vi "Voltage_Current_Sweep.vi"() -> ()   [LabVIEW 2016]
uses:
  <instrlib>/Keithley 24XX/Public/Data/Read (Single Point).vi
  <instrlib>/Keithley 24XX/Keithley 24XX.lvlib
panel:
  in  "Tab Control":enum32{"Voltage", "Current"}(tab)
  in  "Start (V)":dbl
  in  "End (V)":dbl=100.0
  in  "Compliance (V)":dbl=0.1
  in  "Interval (V)":dbl=100.0
  in  "Start (mA)":dbl
  in  "End (mA)":dbl=100.0
  in  "Compliance (A)":dbl=0.1
  in  "Interval (mA)":dbl=100.0
  in  "file (use dialog)":path
  in  "2wire(F)/4wire(T)":bool=TRUE
  out "IV":cluster{dbl[], dbl[]}(graph)
  out "Voltage":sgl=100.0186
  out "Current":sgl=-1.469503e-10
  out "Resistance":sgl=-680628800000.0
  in  "Delay Time (s)":dbl=1.0
  out "VR":cluster{dbl[], dbl[]}(graph)
  out "IR":cluster{dbl[], dbl[]}(graph)
  in  "Enable Resistance Auto Range (T:Enable)":bool=TRUE
  in  "Enable Current Auto Range (T:Enable)":bool=TRUE
  in  "Enable Voltage Auto Range (T:Enable)":bool=TRUE
  in  "Resistance Manual Range (1.0)":dbl=1.0
  in  "Current Manual Range (1.0)":dbl=1.0
  in  "Voltage Manual Range (1.0)":dbl=1.0
  in  "Serial Configuration":T1={"Baud Rate"=9600, "Parity"=0, "Data Bits"=8, "Stop Bits"=10, "Flow Control"=0} {"Flow Control" items=["None", "XON/XOFF", "RTS/CTS", "XON/XOFF & RTS/CTS", "DTR/DSR", "XON/XOFF & DTR/DSR"]; "Stop Bits" items=["1.0"=10, "1.5"=15, "2.0"=20]; "Data Bits" items=["7"=7, "8"=8]; "Parity" items=["None", "Odd", "Even", "Mark", "Space"]; "Baud Rate" items=["300"=300, "600"=600, "1200"=1200, "2400"=2400, "4800"=4800, "9600"=9600, "19200"=19200]}
  in  "VISA resource name":refnum<visa-resource-name>="COM5"
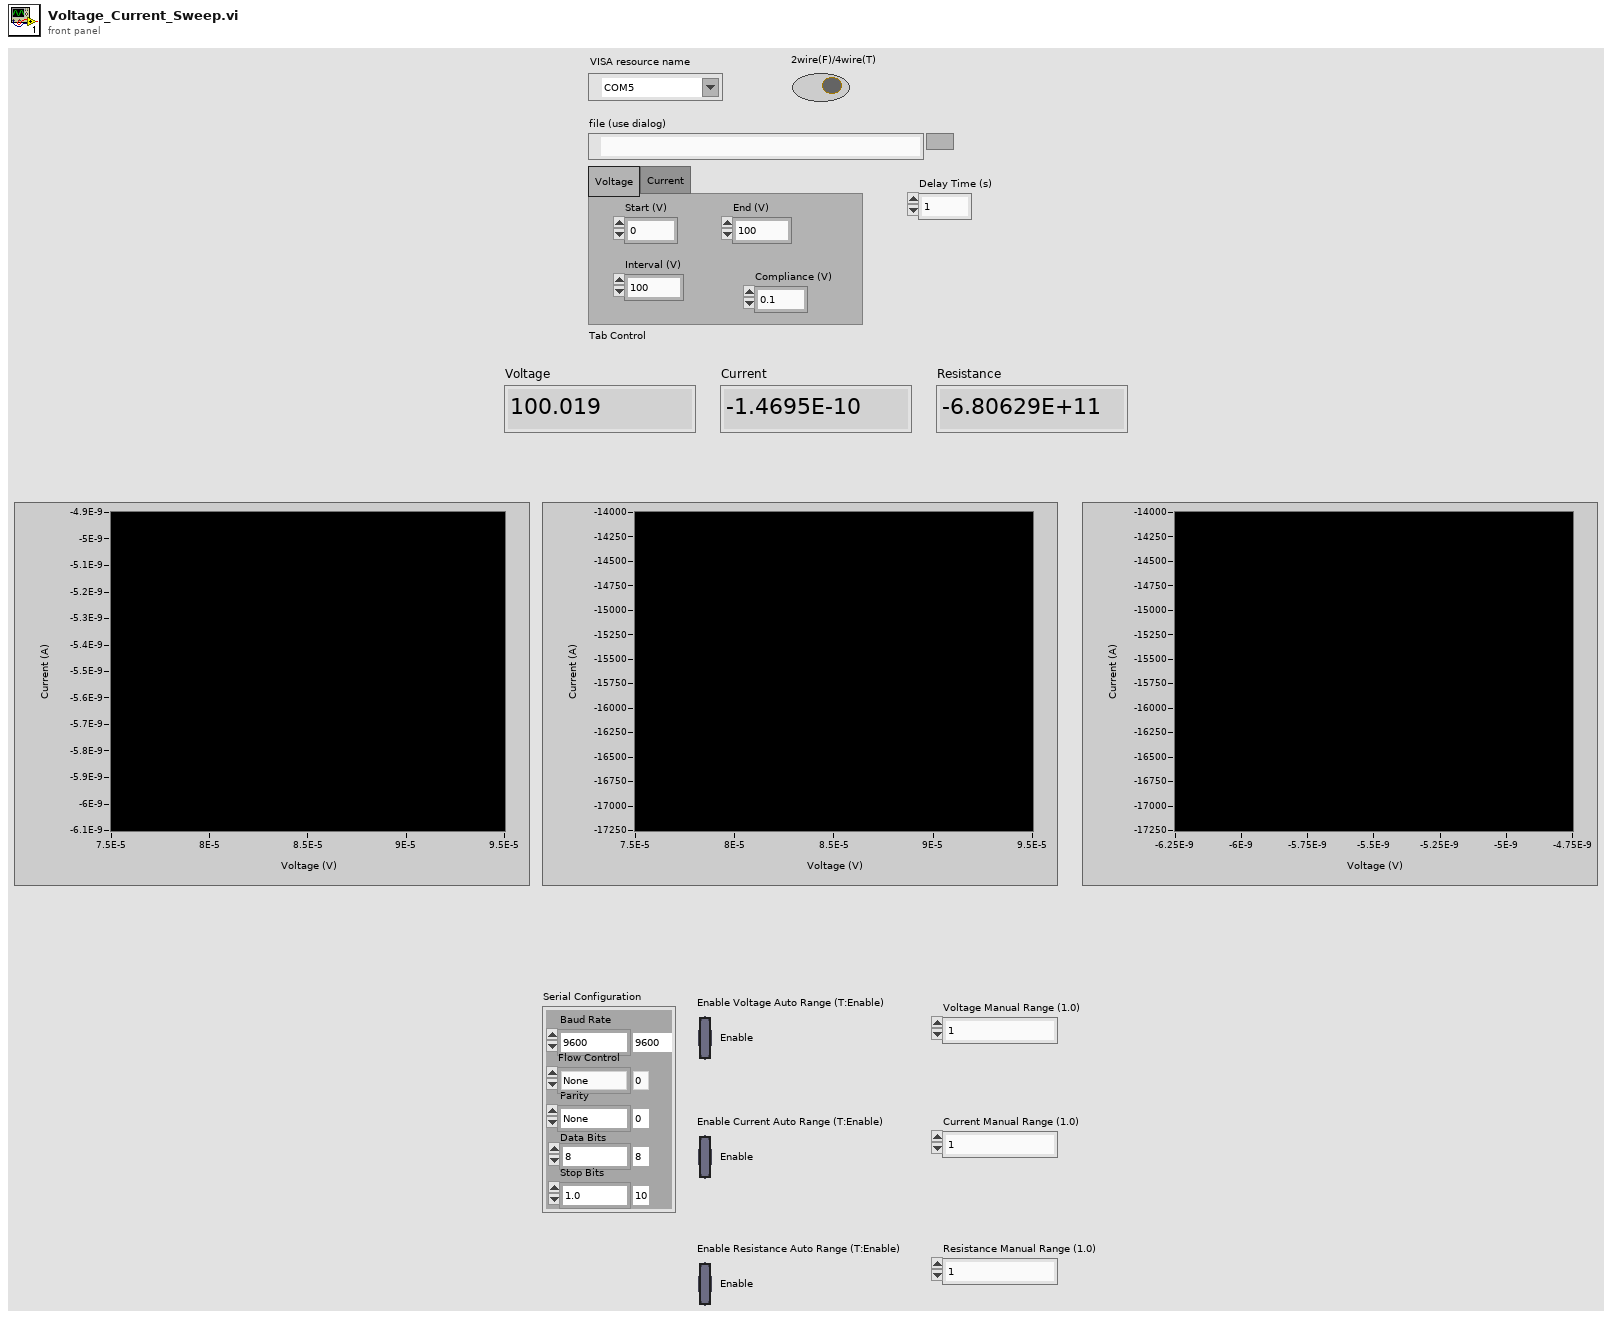
[diagram p1: front panel]
types:
  T1 = cluster{"Baud Rate":u32, "Parity":u16, "Data Bits":u16, "Stop Bits":u16, "Flow Control":u16}
  T2 = enum16{"open", "replace", "create", "open or create", "replace or create", "replace or create with confirmation"}
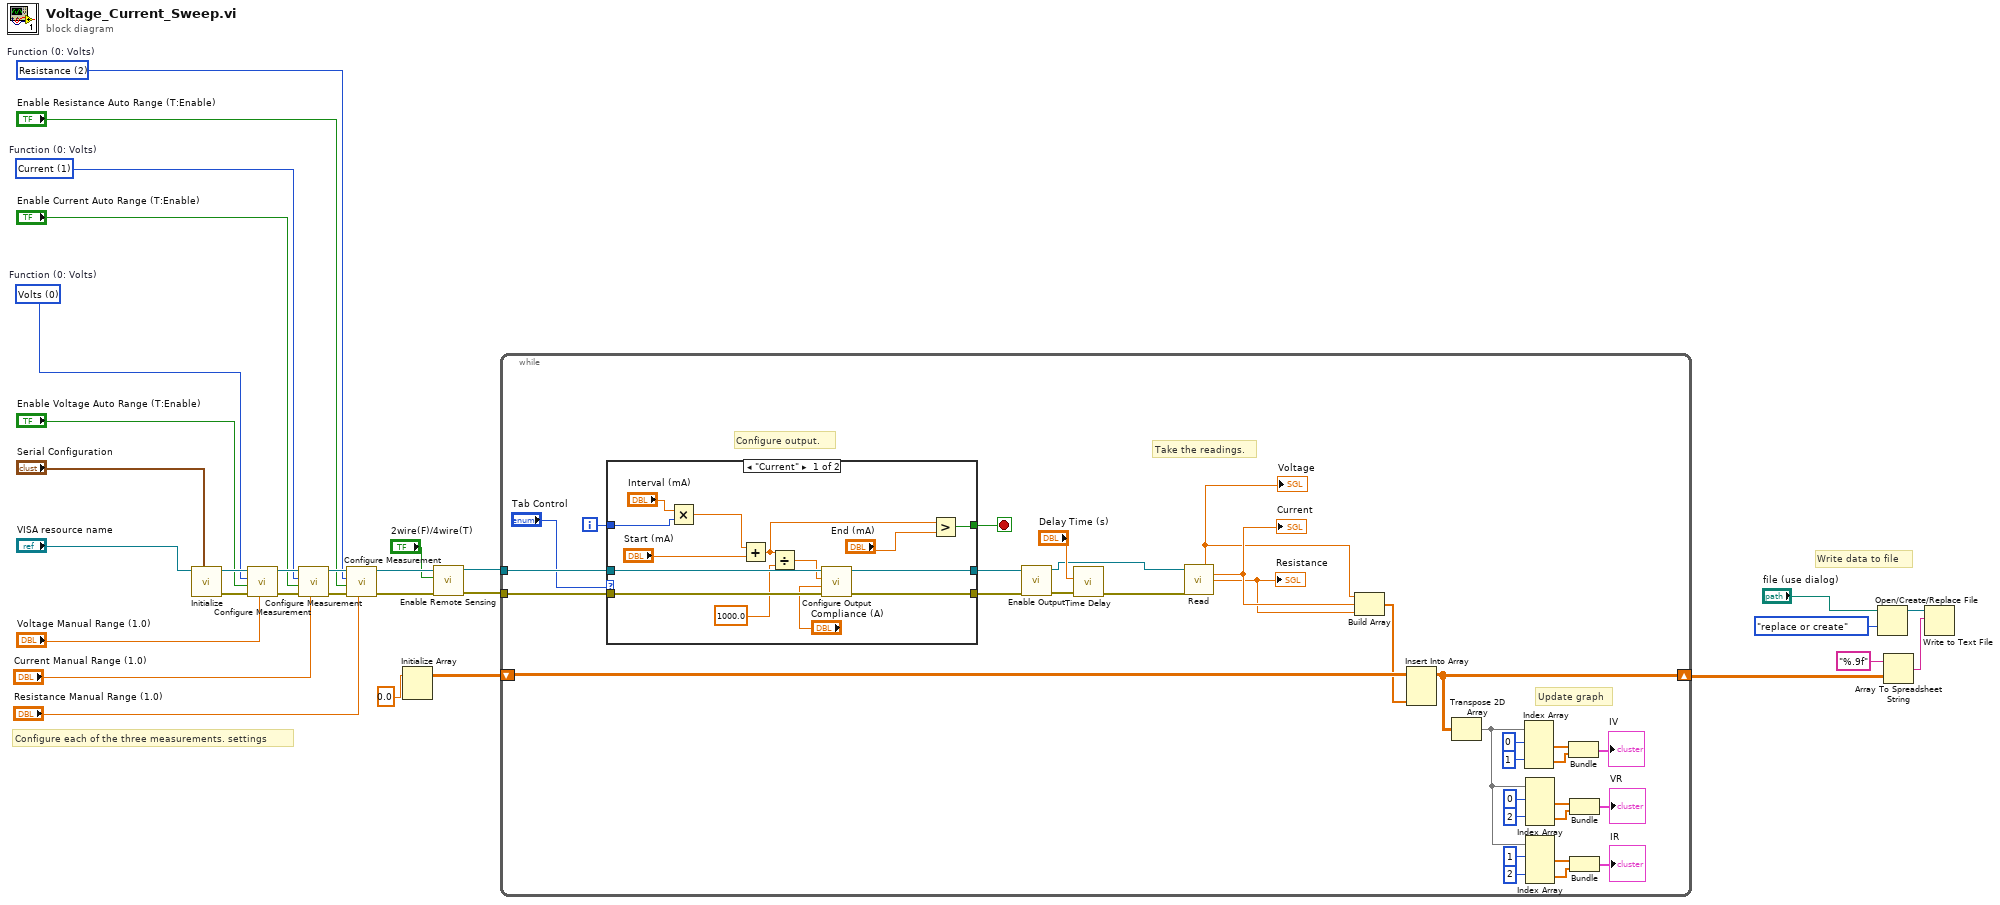
[diagram p0: block diagram]
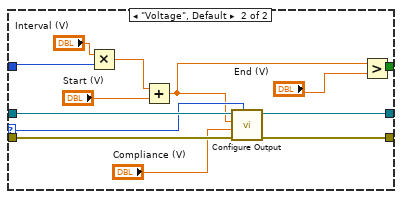
[diagram p2: hidden frame]
diagram:
  w20 = u16 2 items=["Volts", "Current", "Resistance"]  # Function (0: Volts)
  w21 = u16 1 items=["Volts", "Current", "Resistance"]  # Function (0: Volts)
  w22 = u16 0 items=["Volts", "Current", "Resistance"]  # Function (0: Volts)
  # "Write data to file"
  # "Configure each of the three measurements. settings"
  n1 = call <instrlib>:"Initialize.vi"("Serial Configuration"="Serial Configuration", "VISA resource name"="VISA resource name") -> ("error out"=w27:errorcluster, "VISA resource name out"=w28:refnum<visa-resource-name>)  [unwired: 8 in]
  n2 = call <instrlib>:"Configure Measurement.vi"("Manual Range (1.0)"="Voltage Manual Range (1.0)", "error in (no error)"=w27, "Enable Auto Range (T:Enable)"="Enable Voltage Auto Range (T:Enable)", "Function (0: Volts)"=w22, "VISA resource name"=w28) -> ("error out"=w25:errorcluster, "VISA resource name out"=w26:refnum<visa-resource-name>)  [unwired: 5 in]
  n3 = call <instrlib>:"Configure Measurement.vi"("Manual Range (1.0)"="Current Manual Range (1.0)", "error in (no error)"=w25, "Enable Auto Range (T:Enable)"="Enable Current Auto Range (T:Enable)", "Function (0: Volts)"=w21, "VISA resource name"=w26) -> ("error out"=w24:errorcluster, "VISA resource name out"=w23:refnum<visa-resource-name>)  [unwired: 5 in]
  n4 = call <instrlib>:"Configure Measurement.vi"("Manual Range (1.0)"="Resistance Manual Range (1.0)", "error in (no error)"=w24, "Enable Auto Range (T:Enable)"="Enable Resistance Auto Range (T:Enable)", "Function (0: Volts)"=w20, "VISA resource name"=w23) -> ("error out"=w9:errorcluster, "VISA resource name out"=w10:refnum<visa-resource-name>)  [unwired: 5 in]
  n5 = Initialize Array(0.0 ("element")) -> (w11:dbl[][])  [unwired: 2 in]
  n6 = call <instrlib>:"Enable Remote Sensing.vi"("error in (no error)"=w9, "Enable Remote Sensing (T: Enable)"="2wire(F)/4wire(T)", "VISA resource name"=w10) -> ("error out"=w7:errorcluster, "VISA resource name out"=w8:refnum<visa-resource-name>)  [unwired: 7 in]
  n7 = while {
    tunnel: w7 -> [w62]
    tunnel: w8 -> [w63]
    shift-right: [w57] -> w13
    shift-left: w11 -> [w61]
    i -> [w31]
    stop <- w33 stop-if-true
    # "Configure output."
    # "Update graph"
    # "Take the readings."
    n8 = case shown="\"Current\"" "Tab Control" {
      selector: "Tab Control" -> [_ w83]
      tunnel: w63 -> [w77 w90]
      tunnel: w62 -> [w76 w89]
      tunnel: [w74 w87] -> w50
      tunnel: [w73 w86] -> w48
      tunnel: [w69 w84] -> w33
      tunnel: w31 -> [w66 w80]
      frame "Current" {
        n9 = Multiply(x="Interval (mA)", y=w66) -> (x*y=w65:dbl)
        n10 = Add(x=w65, y="Start (mA)") -> (x+y=w68:dbl)
        n11 = Divide(x=w68, y=1000.0) -> (x/y=w70:dbl)
        n12 = call <instrlib>:"Configure Output.vi"("error in (no error)"=w76, "Compliance  Level (0.1)"="Compliance (A)", "Output Level (0)"=w70, "VISA resource name"=w77) -> ("error out"=w73:errorcluster, "VISA resource name out"=w74:refnum<visa-resource-name>)  [unwired: 6 in]
        n13 = Greater?(x=w68, y="End (mA)") -> (0:w69:bool)
      }
      frame "Voltage", Default {
        n14 = Multiply(x="Interval (V)", y=w80) -> (x*y=w79:dbl)
        n15 = Add(x=w79, y="Start (V)") -> (x+y=w78:dbl)
        n16 = call <instrlib>:"Configure Output.vi"("Source Mode  (0: Voltage)"=w83, "error in (no error)"=w89, "Compliance  Level (0.1)"="Compliance (V)", "Output Level (0)"=w78, "VISA resource name"=w90) -> ("error out"=w86:errorcluster, "VISA resource name out"=w87:refnum<visa-resource-name>)  [unwired: 5 in]
        n17 = Greater?(x=w78, y="End (V)") -> (0:w84:bool)
      }
    }
    n18 = call <instrlib>:"Enable Output.vi"("error in (no error)"=w48, "VISA resource name"=w50) -> ("error out"=w47:errorcluster, "VISA resource name out"=w49:refnum<visa-resource-name>)  [unwired: 8 in]
    n19 = call "Time Delay"("error in (no error)"=w47, "Delay Time (s)"="Delay Time (s)") -> ("error out"=w53:errorcluster)  [unwired: 9 in]
    n20 = call-poly <instrlib>:"Read.vi"("VISA resource name"=w49, "error in (no error)"=w53) -> ("Voltage"=w54:sgl, "Current"=w55:sgl, "Resistance"=w51:sgl)  [unwired: 7 in, 4 out]
    "Voltage" <- w54
    "Current" <- w55
    "Resistance" <- w51
    n21 = Build Array(w54, w55, w51) -> (w56:sgl[])
    n22 = Insert Into Array(array=w61, new element=w56) -> (w57:dbl[][])  [unwired: 2 in]
    n23 = Transpose 2D Array(2D array=w57) -> (transposed array=w34:dbl[][])
    n24 = Index Array(array=w34, index (row) #1=0 ("index (row)"), index (row) #2=1 ("index (row)")) -> (element #1=w59:dbl[], element #2=w60:dbl[])  [unwired: 2 in]
    n25 = Index Array(array=w34, index (row) #1=0 ("index (row)"), index (row) #2=2 ("index (row)")) -> (element #1=w43:dbl[], element #2=w44:dbl[])  [unwired: 2 in]
    n26 = Index Array(array=w34, index (row) #1=1 ("index (row)"), index (row) #2=2 ("index (row)")) -> (element #1=w38:dbl[], element #2=w39:dbl[])  [unwired: 2 in]
    n27 = Bundle(w59, w60) -> (→"IV":cluster{dbl[], dbl[]})  [unwired: 1 in]
    n28 = Bundle(w43, w44) -> (→"VR":cluster{dbl[], dbl[]})  [unwired: 1 in]
    n29 = Bundle(w38, w39) -> (→"IR":cluster{dbl[], dbl[]})  [unwired: 1 in]
  }
  n30 = Open/Create/Replace File(file path (use dialog)="file (use dialog)", operation (0:open)=T2."replace or create") -> (refnum out=w2:refnum<file>)  [unwired: 4 in, 2 out]
  n31 = Array To Spreadsheet String(array=w13, 3:"%.9f" ("format string")) -> (spreadsheet string=w5:string)  [unwired: 1 in]
  n32 = Write to Text File(file (use dialog)=w2, text=w5) -> ()  [unwired: 2 in, 3 out]
